vi "Layout Subpanels.vi"(8 "error in (no error)":errorcluster, 9 "SubPanels in":refnum<vi>[](array[refnum]), 10 "Panels in":refnum<class "ArrayPanel.lvclass">[][](array[class]), 11 "2DArrayManager in":refnum<class "2DArrayManager.lvclass">) -> (0 "error out":errorcluster, 1 "SubPanels":refnum<vi>[](array[refnum]), 2 "Used Count":i32, 3 "2DArrayManager out":refnum<class "2DArrayManager.lvclass">, 5 "Insufficient Subpanels":bool)   [LabVIEW 2020, in "OOPanel.lvlib" / "2DArrayManager.lvclass"]
uses:
  2DArrayManager.lvclass
  2DArrayManager.lvclass/2DArrayManager.ctl
  Manager/Manager.lvclass
  ArrayPanel/ArrayPanel.lvclass
  C:/dev/lv20CE/lv-oopanel/OOPanel/Panel/Panel.lvclass
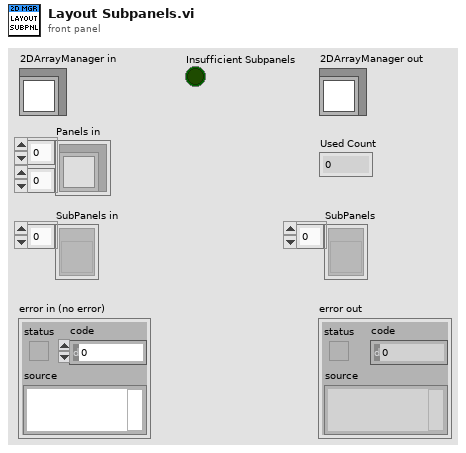
[diagram p1: front panel]
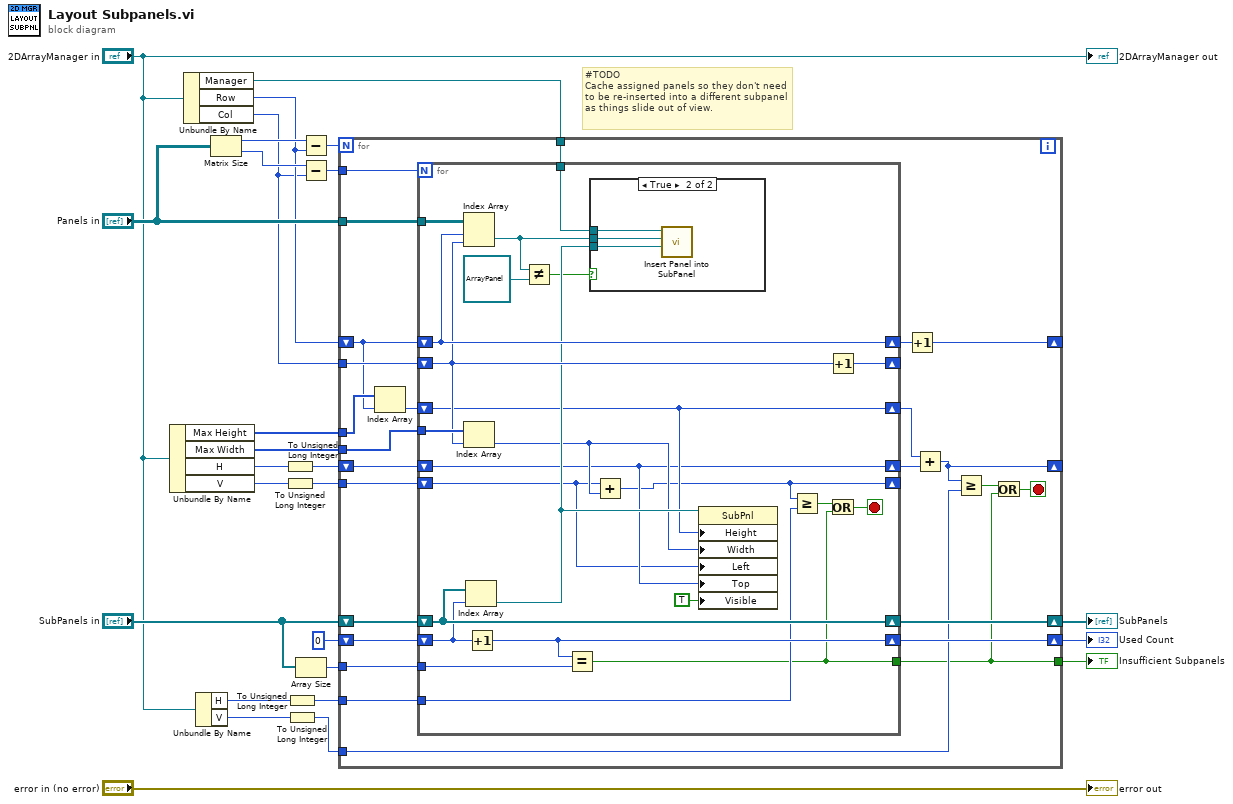
[diagram p0: block diagram]
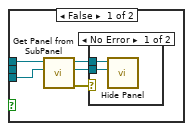
[diagram p2: hidden frame]
diagram:
  # "#TODO\nCache assigned panels so they don't need to be re-inserted into a different subpanel as things slide out of view."
  n1 = Unbundle By Name("2DArrayManager in") -> ("Max Height"=w10:u32[], "Max Width"=w9:u32[], "H"=w12:i32, "V"=w11:i32)
  n2 = Unbundle By Name("2DArrayManager in") -> ("Manager"=w20:refnum<class "Manager.lvclass">, "Row"=w15:i32, "Col"=w13:i32)
  n3 = Unbundle By Name("2DArrayManager in") -> ("H"=w5:i32, "V"=w4:i32)
  n4 = Matrix Size(0:"Panels in") -> (1:w25:i32, 2:w23:i32)
  n5 = To Unsigned Long Integer(number=w12) -> (unsigned 32bit integer=w8:u32)
  n6 = To Unsigned Long Integer(number=w11) -> (unsigned 32bit integer=w7:u32)
  n7 = To Unsigned Long Integer(number=w5) -> (unsigned 32bit integer=w2:u32)
  n8 = To Unsigned Long Integer(number=w4) -> (unsigned 32bit integer=w3:u32)
  n9 = Array Size(array="SubPanels in") -> (size(s)=w16:i32)
  n10 = Subtract(x=w25, y=w15) -> (x-y=w24:i32)
  n11 = Subtract(x=w23, y=w13) -> (x-y=w22:i32)
  n12 = for {
    N: w24 -> [_]
    tunnel: w22 -> [w51]
    tunnel: "Panels in" -> [w50]
    tunnel: w20 -> [w49]
    shift-right: [w47] -> w19
    shift-left: "SubPanels in" -> [w48]
    shift-right: [w42] -> w14
    shift-left: 0 -> [w46]
    tunnel: w16 -> [w45]
    tunnel: [w28] -> w1
    shift-right: [w43] -> _
    shift-left: w15 -> [w36]
    tunnel: w13 -> [w41]
    shift-right: [w31] -> _
    shift-left: w8 -> [w40]
    tunnel: w10 -> [w37]
    tunnel: w9 -> [w38]
    tunnel: w7 -> [w39]
    tunnel: w2 -> [w32]
    tunnel: w3 -> [w30]
    stop <- w27 stop-if-true
    n13 = Index Array(array=w37, index=w36) -> (element=w35:u32)
    n14 = for {
      N: w51 -> [_]
      tunnel: w50 -> [w75]
      tunnel: w49 -> [w74]
      shift-right: [w73] -> w47
      shift-left: w48 -> [w73]
      shift-right: [w70] -> w42
      shift-left: w46 -> [w72]
      tunnel: w45 -> [w71]
      tunnel: [w57] -> w28
      shift-right: [w68] -> w44
      shift-left: w36 -> [w68]
      shift-right: [w69] -> _
      shift-left: w41 -> [w66]
      shift-right: [w62] -> w34
      shift-left: w40 -> [w62]
      shift-right: [w61] -> _
      shift-left: w39 -> [w59]
      tunnel: w38 -> [w67]
      shift-right: [w64] -> w33
      shift-left: w35 -> [w64]
      tunnel: w32 -> [w60]
      stop <- w56 stop-if-true
      n15 = Index Array(array=w75, index (row)=w68, index (col)=w66) -> (element=w54:refnum<class "ArrayPanel.lvclass">)
      n16 = Index Array(array=w67, index=w66) -> (element=w63:u32)
      n17 = Index Array(array=w73, index=w72) -> (element=w65:refnum<vi>)
      n18 = Increment(x=w72) -> (x+1=w70:i32)
      n19 = Not Equal?(x=w54, y=refnum<class "ArrayPanel.lvclass"> refnum) -> (x != y?=w52:bool)
      n20 = Equal?(x=w70, y=w71) -> (x = y?=w57:bool)
      n21 = case shown="True" w52 {
        tunnel: w74 -> [w80 w85]
        tunnel: w65 -> [w79 w84]
        tunnel: w54 -> [_ w83]
        frame False {
          n22 = call "Get Panel from SubPanel.vi"("SubPanel"=w79, "Manager in"=w80) -> ("error out"=w76:errorcluster, "Panel"=w77:refnum<class "Panel.lvclass">, "Manager out"=w78:refnum<class "Manager.lvclass">)  [unwired: 6 in, 1 out]
          n23 = case shown="No Error" w76 {
            tunnel: w78 -> [w82 _]
            tunnel: w77 -> [w81 _]
            frame No Error {
              n24 = call "Hide Panel.vi"("Panel In"=w81, "Manager in"=w82) -> ()  [unwired: 7 in, 3 out]
            }
            frame Error {
            }
          }
        }
        frame True {
          n25 = call "Insert Panel into SubPanel.vi"("SubPanel"=w84, "Panel In"=w83, "Manager in"=w85) -> ()  [unwired: 6 in, 3 out]
        }
      }
      n26 = Add(x=w59, y=w63) -> (x+y=w61:u32)
      n27 = property class="SubPnl"(reference=w65, "Height"=w64, "Width"=w63, "Left"=w59, "Top"=w62, "Visible"=TRUE) -> ()  [unwired: 1 in, 2 out]
      n28 = Greater Or Equal?(x=w61, y=w60) -> (x >= y?=w58:bool)
      n29 = Increment(x=w66) -> (x+1=w69:i32)
      n30 = Or(x=w58, y=w57) -> (x .or. y?=w56:bool)
    }
    n31 = Increment(x=w44) -> (x+1=w43:i32)
    n32 = Add(x=w33, y=w34) -> (x+y=w31:u32)
    n33 = Greater Or Equal?(x=w31, y=w30) -> (x >= y?=w29:bool)
    n34 = Or(x=w29, y=w28) -> (x .or. y?=w27:bool)
  }
  "Used Count" <- w14
  "SubPanels" <- w19
  "Insufficient Subpanels" <- w1
  "error out" <- "error in (no error)"
  "2DArrayManager out" <- "2DArrayManager in"
